vi "PROJECT.vi"() -> ()   [LabVIEW 2020]
uses:
  <vilib>/Utility/file.llb/Read Delimited Spreadsheet (string).vi
  <vilib>/Utility/file.llb/Read Delimited Spreadsheet (DBL).vi
  <vilib>/Utility/file.llb/Write Delimited Spreadsheet (DBL).vi
panel:
  out "TOTAL EVENTS":dbl
  out "USD TO RM":dbl
  out "CRUDE OIL":dbl
  out "TIME":string
  out "DATE":string
  out "EVENT REPORT":string[][](array[string])
  out "INDICATOR":T1
  in  "SECURITY":T2 {"TEMPERATURE" scale=27.0..110.0}
  out "ITEM RECEIVED":bool
  out "PICKUP 4":dbl(slide) scale=0.0..10.0
  out "PROCESSTROLLEYVER 3":dbl(slide)
  out "PICKUP 3":dbl(slide) scale=0.0..10.0
  out "PICKUP 2":dbl(slide) scale=0.0..10.0
  out "PROCESSTROLLEYVER 2":dbl(slide) scale=0.0..10.0
  out "PROCESSTROLLEYVER":dbl(slide) scale=0.0..10.0
  out "BOXVERT":dbl(slide) scale=0.0..10.0
  out "PICKUP":i32(slide) scale=0.0..10.0
  out "TINY":bool
  out "SMALL":bool
  out "MEDIUM":bool
  out "BIG":bool
  out "PRODUCT AVAILABLITY":bool=TRUE
  out "Boolean 2":bool
  out "Boolean":bool
  out "index of element":i32
  out "PRODUCT NOT AVAILABLE":bool
  out "Start":dbl(slide) scale=0.0..10.0
  out "PATH1":dbl(slide) scale=0.0..10.0
  out "PATH7":dbl(slide) scale=0.0..10.0
  out "PATH4":dbl(slide) scale=0.0..10.0
  out "PATH 3":dbl(slide)
  out "PATH9":dbl(slide) scale=0.0..10.0
  out "PATH8":dbl(slide)
  out "PATH2":dbl(slide) scale=0.0..10.0
  out "PATH6":dbl(slide)
  out "PATH5":dbl(slide)
  out "PATH12":dbl(slide) scale=0.0..10.0
  out "PATH11":dbl(slide) scale=0.0..10.0
  out "PATH10":dbl(slide) scale=0.0..10.0
  out "BIG BOX":dbl(slide) scale=0.0..10.0
  out "PACKAGING":dbl(slide) scale=0.0..10.0
  out "x+1":dbl
  out "ALARM":dbl
  out "PROCESSING OFF":bool
  out "login":bool
  out "STRING":string
  out "WEIGHT":string
  out "BOXTYPE":string
  out "ORDER ID":string
  out "all rows":string[](array[string])
  # "MARKET INFORMATION"
  # "AUTOMATED WAREHOUSE MANAGEMENT SYSTEM\n                                                          -NI LABVIEW \n                                                                 -BY ABHISHEK KUMAR JHA"
  # "MEDIUM"
  # "PROCESSING HOUSE"
  # "TINY"
  # "SMALL"
  # "BIG"
  # "SECURITY AND ALARM CENTER"
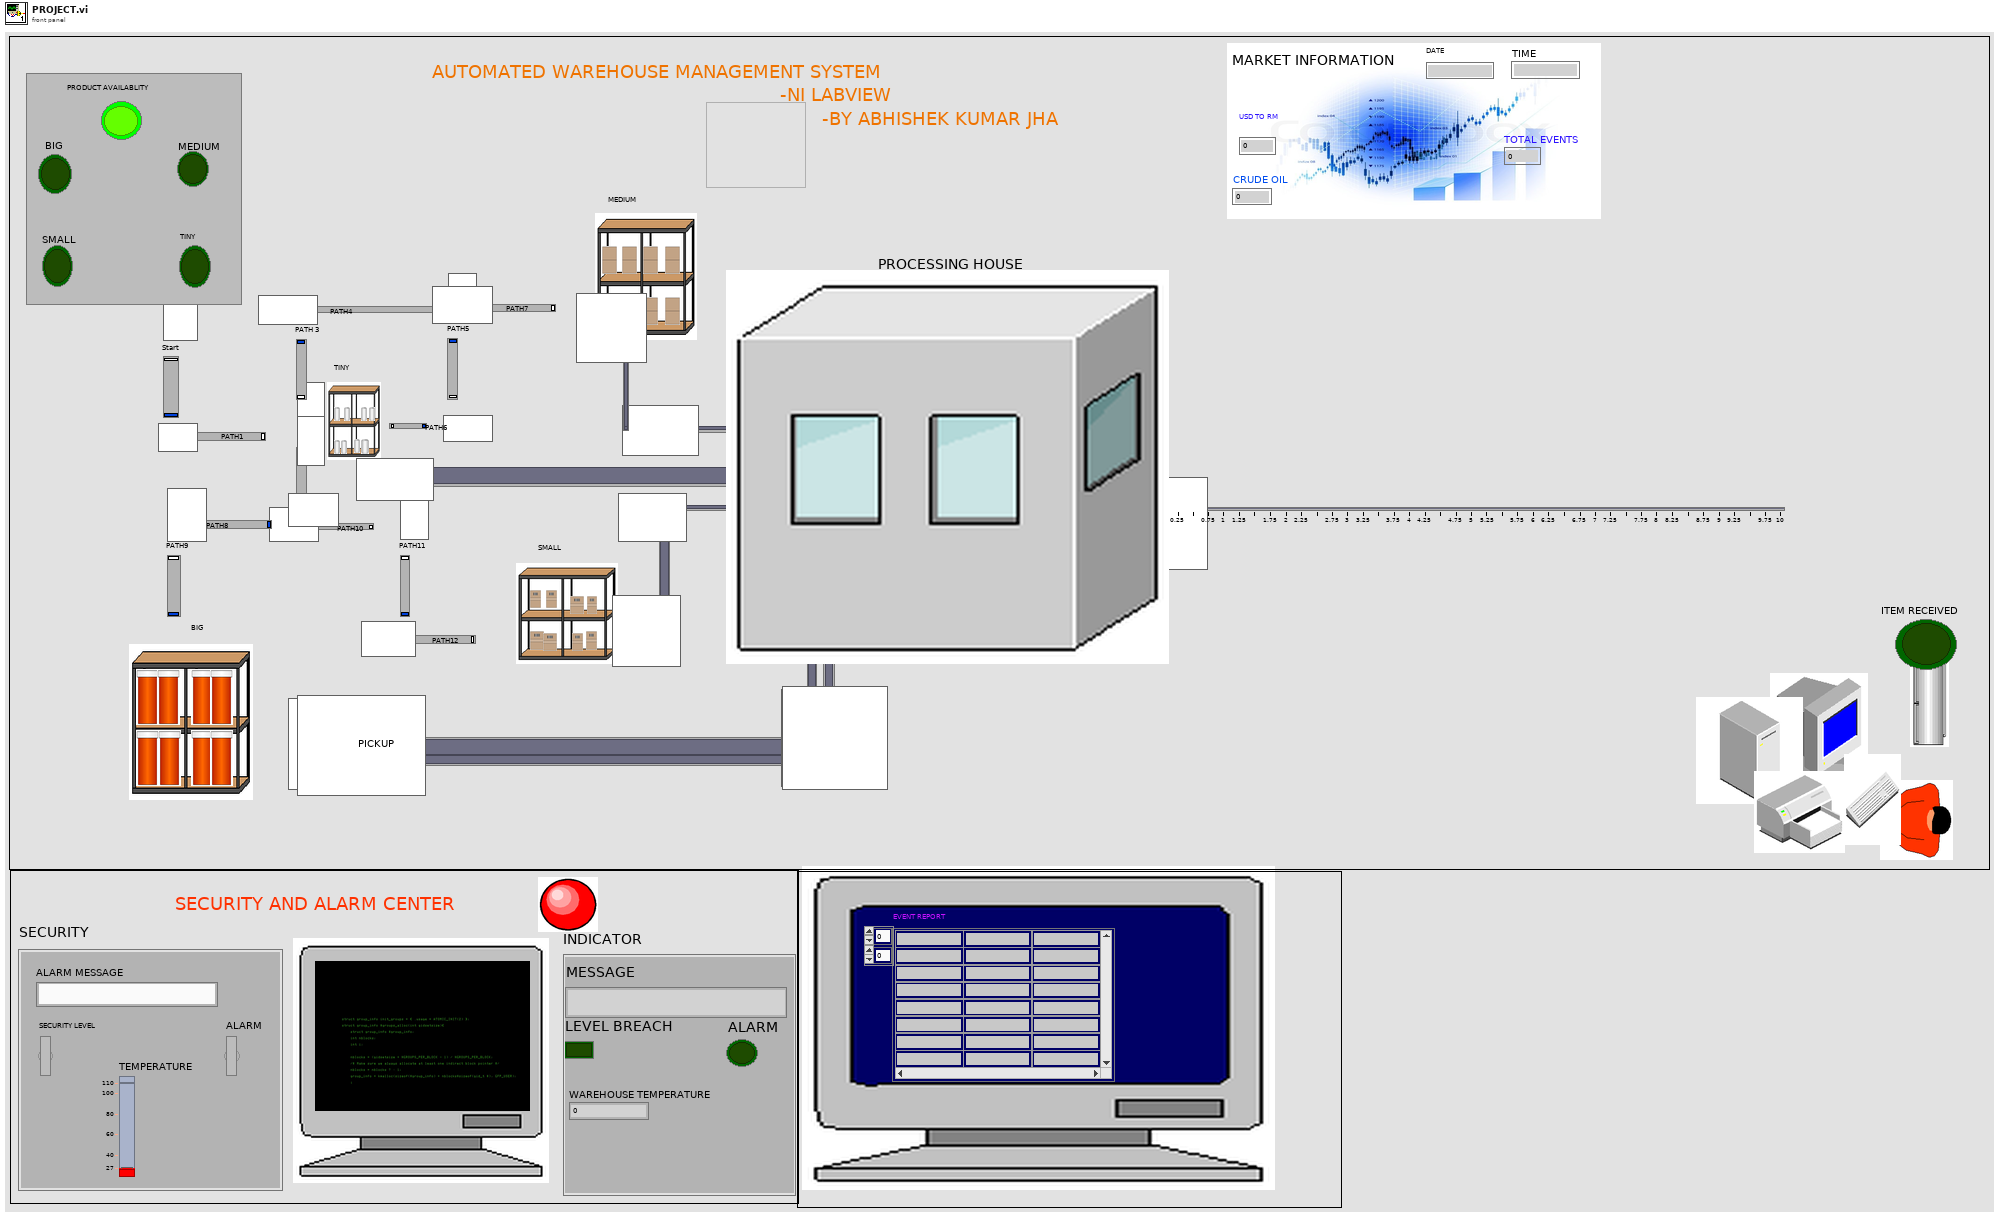
[diagram p1: front panel]
types:
  T1 = cluster{"MESSAGE":string, "LEVEL BREACH":bool, "ALARM":bool, "WAREHOUSE TEMPERATURE":dbl}
  T2 = cluster{"ALARM MESSAGE":string, "SECURITY LEVEL":bool, "ALARM":bool, "TEMPERATURE":dbl}
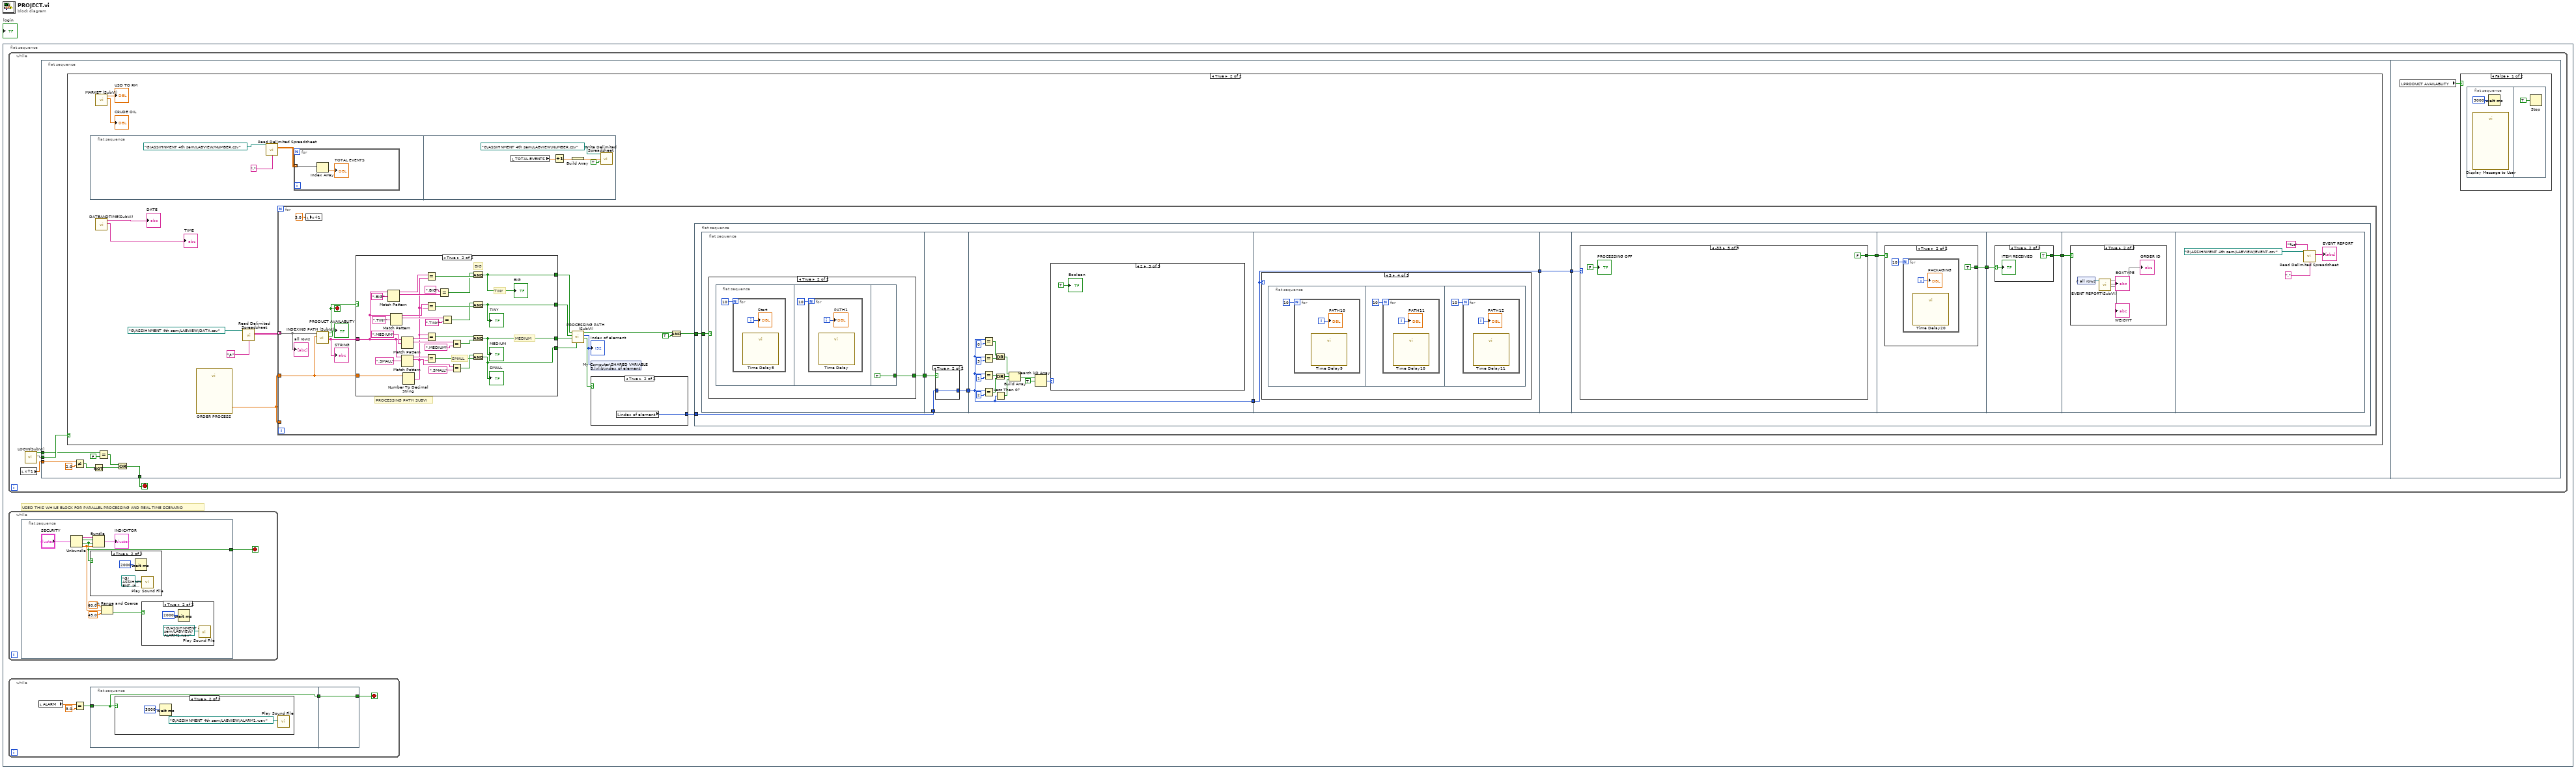
[diagram p0: block diagram]
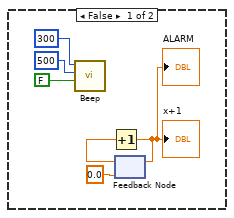
[diagram p5: hidden frame]
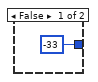
[diagram p6: hidden frame]
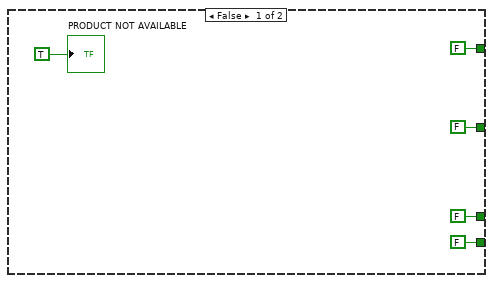
[diagram p7: hidden frame]
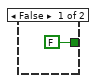
[diagram p8: hidden frame]
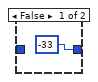
[diagram p9: hidden frame]
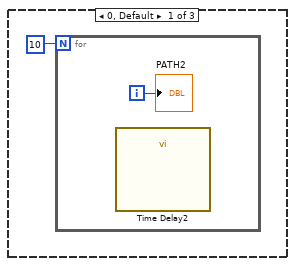
[diagram p10: hidden frame]
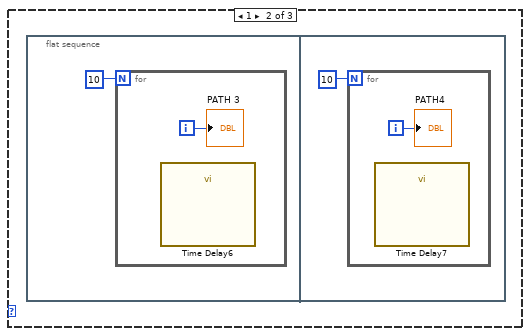
[diagram p11: hidden frame]
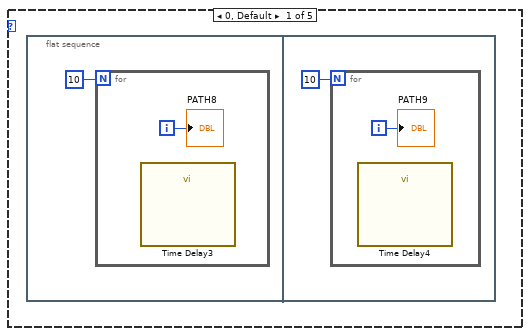
[diagram p12: hidden frame]
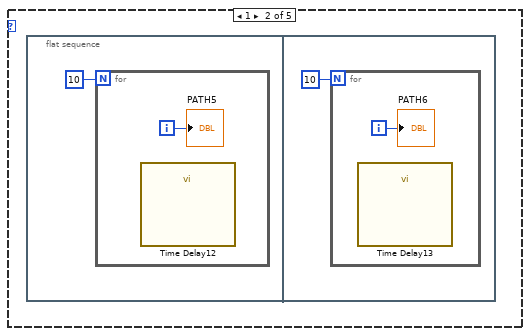
[diagram p13: hidden frame]
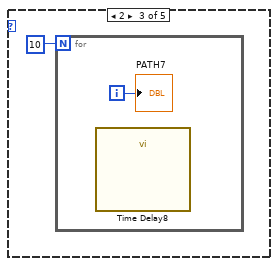
[diagram p14: hidden frame]
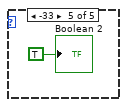
[diagram p15: hidden frame]
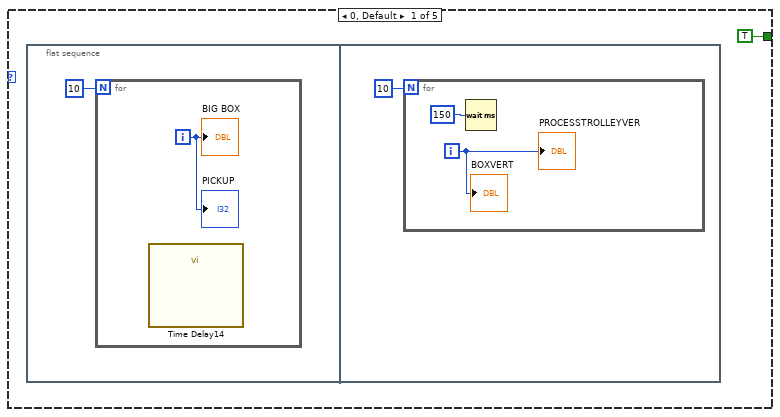
[diagram p16: hidden frame]
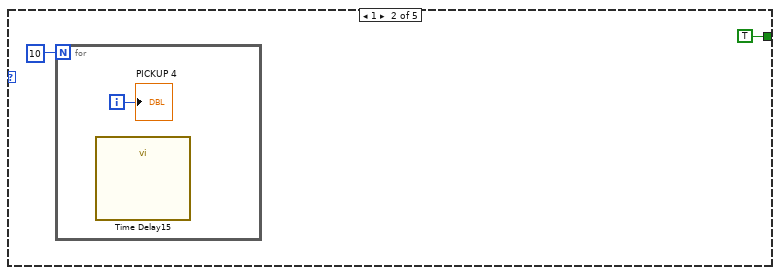
[diagram p17: hidden frame]
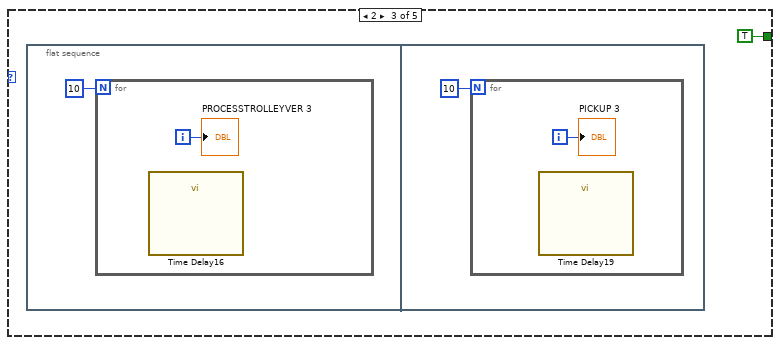
[diagram p18: hidden frame]
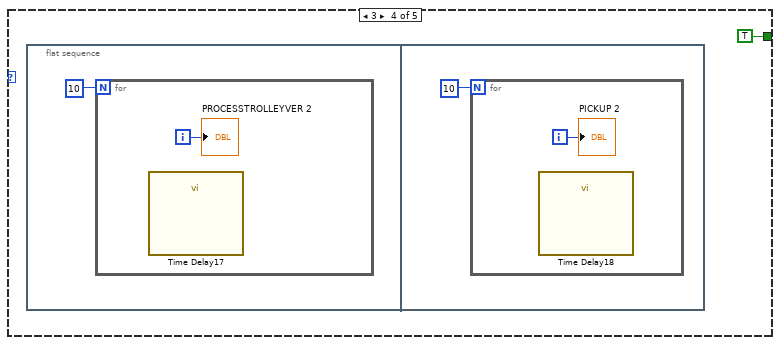
[diagram p19: hidden frame]
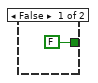
[diagram p20: hidden frame]
diagram:
  n1 = flat-sequence {
    frame #0 {
      # "USED THIS WHILE BLOCK FOR PARALLEL PROCESSING AND REAL TIME SCENARIO"
      n2 = while {
        stop <- w25 stop-if-true
        n3 = local read "x+1"() -> (w27:dbl)
        n4 = call "LOGIN(SubVI).vi"() -> (2:w26, "Boolean"=w24:bool)  [unwired: 10 in]
        n5 = flat-sequence {
          tunnel: w27 -> [w34]
          tunnel: w26 -> [w33]
          tunnel: [w29] -> w25
          tunnel: w24 -> [w28]
          frame #0 {
            n6 = case shown="True" w33 {
              frame False {
                n7 = call <vilib>:"Beep.vi"("use system alert? (T)"=FALSE, "duration (msec)"=u32 500, "frequency (Hz)"=u32 300) -> ()  [unwired: 9 in]
                n8 = feedback #1(0.0) -> (w42:dbl)
                n9 = Increment(x=w42) -> (x+1=w41:dbl)
                "x+1" <- w41
                "ALARM" <- w41
                n10 = feedback-in #1(w41) -> ()
              }
              frame True {
                n11 = flat-sequence {
                  frame #0 {
                    n12 = call-poly <vilib>:"Read Delimited Spreadsheet.vi"("file path (dialog if empty)"=path "G:/ASSIHNMENT 4th sem/LABVIEW/NUMBER.csv", "delimiter (\\t)"="," ("delimiter (\\t)")) -> ("all rows"=w51:dbl[][])  [unwired: 8 in, 5 out]
                    n13 = for {
                      tunnel: w51 -> [w55] mode=indexing
                      n14 = Index Array(array=w55) -> (element=→"TOTAL EVENTS":dbl)  [unwired: 1 in]
                    }
                  }
                  frame #1 {
                    n15 = local read "TOTAL EVENTS"() -> (w57:dbl)
                    n16 = Increment(x=w57) -> (x+1=w56:dbl)
                    n17 = Build Array(w56) -> (w58:dbl[])
                    n18 = call-poly <vilib>:"Write Delimited Spreadsheet.vi"("file path (dialog if empty)"=path "G:/ASSIHNMENT 4th sem/LABVIEW/NUMBER.csv", "1D data"=w58, "append to file? (new file:F)"=TRUE) -> ()  [unwired: 11 in, 2 out]
                  }
                }
                n19 = call "MARKET (SubVI).vi"() -> ("CRUDE OIL"=→"CRUDE OIL":dbl, "USD TO RM"=→"USD TO RM":dbl)  [unwired: 10 in]
                n20 = call "DATEANDTIME(SubVI).vi"() -> ("TIME"=→"TIME":string, "DATE"=→"DATE":string)  [unwired: 10 in]
                n21 = call "ORDER PROCESS"() -> ("ORDER ID:-"=w47:dbl)  [unwired: 17 in, 2 out]
                n22 = call-poly <vilib>:"Read Delimited Spreadsheet.vi"("file path (dialog if empty)"=path "G:/ASSIHNMENT 4th sem/LABVIEW/DATA.csv", "delimiter (\\t)"="\t," ("delimiter (\\t)")) -> ("all rows"=w48:string[][])  [unwired: 8 in, 5 out]
                n23 = for {
                  tunnel: w48 -> [w65] mode=indexing
                  tunnel: w47 -> [w66]
                  tunnel: w47 -> [_]
                  stop <- w75 stop-if-true
                  # "PROCESSING PATH SUBVI"
                  n24 = local write "x+1"(3.0 ("x+1")) -> ()
                  n25 = call "INDEXING PATH (SubVI).vi"("ORDER ID:-"=w66, "ROWS"=w65) -> ("STRING"=w76:string, "PRODUCT AVAILABLITY"=→"PRODUCT AVAILABLITY":bool, "INDIDCATOR"=w75:bool)  [unwired: 7 in]
                  "STRING" <- w76
                  n26 = case shown="True" w75 {
                    tunnel: w66 -> [_ w111]
                    tunnel: w76 -> [_ w88]
                    tunnel: [FALSE ("Boolean 2") w87] -> w74
                    tunnel: [FALSE w86] -> w73
                    tunnel: [FALSE w85] -> w72
                    tunnel: [FALSE w84] -> w71
                    frame False {
                      "PRODUCT NOT AVAILABLE" <- TRUE ("PRODUCT NOT AVAILABLE")
                    }
                    frame True {
                      # "BIG"
                      # "TINY"
                      # "MEDIUM"
                      # "SMALL"
                      n27 = Match Pattern(string=w88, regular expression=",BIG") -> (before substring=w110:string, match substring=w113:string)  [unwired: 1 in, 2 out]
                      n28 = Match Pattern(string=w88, regular expression=",TINY") -> (before substring=w92:string, match substring=w103:string)  [unwired: 1 in, 2 out]
                      n29 = Match Pattern(string=w88, regular expression=",MEDIUM") -> (before substring=w98:string, match substring=w104:string)  [unwired: 1 in, 2 out]
                      n30 = Match Pattern(string=w88, regular expression=",SMALL") -> (before substring=w95:string, match substring=w102:string)  [unwired: 1 in, 2 out]
                      n31 = Number To Decimal String(number=w111) -> (decimal integer string=w91:string)  [unwired: 1 in]
                      n32 = Equal?(x=w110, y=w91) -> (x = y?=w109:bool)
                      n33 = Equal?(x=w92, y=w91) -> (x = y?=w90:bool)
                      n34 = Equal?(x=w91, y=w98) -> (x = y?=w97:bool)
                      n35 = Equal?(x=w95, y=w91) -> (x = y?=w94:bool)
                      n36 = Equal?(x=",BIG", y=w113) -> (x = y?=w108:bool)
                      n37 = Equal?(x=w103, y=",TINY") -> (x = y?=w89:bool)
                      n38 = Equal?(x=w104, y=",MEDIUM") -> (x = y?=w96:bool)
                      n39 = Equal?(x=w102, y=",SMALL") -> (x = y?=w93:bool)
                      n40 = And(x=w108, y=w109) -> (x .and. y?=w87:bool)
                      "BIG" <- w87
                      n41 = And(x=w89, y=w90) -> (x .and. y?=w86:bool)
                      "TINY" <- w86
                      n42 = And(x=w97, y=w96) -> (x .and. y?=w85:bool)
                      "MEDIUM" <- w85
                      n43 = And(x=w93, y=w94) -> (x .and. y?=w84:bool)
                      "SMALL" <- w84
                    }
                  }
                  n44 = call "PROCESSING PATH (SubVI).vi"("Boolean 3"=w71, "Boolean 4"=w72, "Boolean 5"=w73, "Boolean 6"=w74) -> ("Boolean"=w64:bool, "index of element"=w63:i32, "Boolean 2"=w68:bool)  [unwired: 5 in]
                  "index of element" <- w63
                  n45 = shared-variable "My Computer\\SHARED VARIABLE 3.lvlib\\index of element"(w63) -> ()  [unwired: 1 in, 1 out]
                  n46 = case shown="True" w64 {
                    tunnel: [-33 w78] -> w67
                    frame False {
                    }
                    frame True {
                      n47 = local read "index of element"() -> (w78:i32)
                    }
                  }
                  n48 = And(x=w68, y=TRUE) -> (x .and. y?=w69:bool)
                  n49 = flat-sequence {
                    tunnel: w69 -> [w122]
                    tunnel: w67 -> [w120]
                    frame #0 {
                      n50 = flat-sequence {
                        tunnel: w122 -> [w126]
                        tunnel: [w125] -> w121
                        tunnel: [w136] -> w123
                        tunnel: w121 -> [w135]
                        tunnel: w120 -> [w134]
                        tunnel: [w139] -> w124
                        tunnel: w123 -> [w139]
                        tunnel: w124 -> [w161]
                        tunnel: [w161] -> w118
                        tunnel: [w179] -> w119
                        tunnel: w118 -> [w179]
                        tunnel: w119 -> [w181]
                        tunnel: [w180] -> w117
                        tunnel: w117 -> [w204]
                        tunnel: [w203] -> w116
                        tunnel: w116 -> [w209]
                        tunnel: [w210] -> w115
                        tunnel: w115 -> [w214]
                        frame #0 {
                          n51 = case shown="True" w126 {
                            tunnel: [FALSE w128] -> w125
                            frame False {
                            }
                            frame True {
                              n52 = flat-sequence {
                                tunnel: [TRUE] -> w128
                                frame #0 {
                                n53 = for {
                                N: 10 -> [_]
                                i -> [w130]
                                n54 = call "Time Delay5"() -> ()  [unwired: 11 in, 1 out]
                                "Start" <- w130
                                }
                                }
                                frame #1 {
                                n55 = for {
                                N: 10 -> [_]
                                i -> [w132]
                                n56 = call "Time Delay"() -> ()  [unwired: 11 in, 1 out]
                                "PATH1" <- w132
                                }
                                }
                                frame #2 {
                                }
                              }
                            }
                          }
                        }
                        frame #1 {
                          n57 = case shown="True" w135 {
                            tunnel: [-33 w138] -> w136
                            tunnel: w134 -> [_ w138]
                            frame False {
                            }
                            frame True {
                            }
                          }
                        }
                        frame #2 {
                          n58 = Equal?(x=w139, y=0) -> (x = y?=w151:bool)
                          n59 = Equal?(x=w139, y=3) -> (x = y?=w150:bool)
                          n60 = Equal?(x=w139, y=1) -> (x = y?=w147:bool)
                          n61 = Equal?(x=w139, y=2) -> (x = y?=w146:bool)
                          n62 = Or(x=w151, y=w150) -> (x .or. y?=w145:bool)
                          n63 = Or(x=w147, y=w146) -> (x .or. y?=w144:bool)
                          n64 = Less Than 0?(x=w139) -> (x < 0?=w143:bool)
                          n65 = Build Array(w145, w144, w143) -> (w142:bool[])
                          n66 = Search 1D Array(1D array=w142, element=TRUE) -> (index of element=w140:i32)  [unwired: 1 in]
                          n67 = case shown="2" w140 {
                            frame 0, Default {
                              n68 = for {
                                N: 10 -> [_]
                                i -> [w155]
                                n69 = call "Time Delay2"() -> ()  [unwired: 11 in, 1 out]
                                "PATH2" <- w155
                              }
                            }
                            frame 1 {
                              n70 = flat-sequence {
                                frame #0 {
                                n71 = for {
                                N: 10 -> [_]
                                i -> [w157]
                                n72 = call "Time Delay6"() -> ()  [unwired: 11 in, 1 out]
                                "PATH 3" <- w157
                                }
                                }
                                frame #1 {
                                n73 = for {
                                N: 10 -> [_]
                                i -> [w159]
                                n74 = call "Time Delay7"() -> ()  [unwired: 11 in, 1 out]
                                "PATH4" <- w159
                                }
                                }
                              }
                            }
                            frame 2 {
                              "Boolean" <- TRUE
                            }
                          }
                        }
                        frame #3 {
                          n75 = case shown="3" w161 {
                            frame 0, Default {
                              n76 = flat-sequence {
                                frame #0 {
                                n77 = for {
                                N: 10 -> [_]
                                i -> [w163]
                                n78 = call "Time Delay3"() -> ()  [unwired: 11 in, 1 out]
                                "PATH8" <- w163
                                }
                                }
                                frame #1 {
                                n79 = for {
                                N: 10 -> [_]
                                i -> [w165]
                                n80 = call "Time Delay4"() -> ()  [unwired: 11 in, 1 out]
                                "PATH9" <- w165
                                }
                                }
                              }
                            }
                            frame 1 {
                              n81 = flat-sequence {
                                frame #0 {
                                n82 = for {
                                N: 10 -> [_]
                                i -> [w167]
                                n83 = call "Time Delay12"() -> ()  [unwired: 11 in, 1 out]
                                "PATH5" <- w167
                                }
                                }
                                frame #1 {
                                n84 = for {
                                N: 10 -> [_]
                                i -> [w169]
                                n85 = call "Time Delay13"() -> ()  [unwired: 11 in, 1 out]
                                "PATH6" <- w169
                                }
                                }
                              }
                            }
                            frame 2 {
                              n86 = for {
                                N: 10 -> [_]
                                i -> [w171]
                                n87 = call "Time Delay8"() -> ()  [unwired: 11 in, 1 out]
                                "PATH7" <- w171
                              }
                            }
                            frame 3 {
                              n88 = flat-sequence {
                                frame #0 {
                                n89 = for {
                                N: 10 -> [_]
                                i -> [w173]
                                n90 = call "Time Delay9"() -> ()  [unwired: 11 in, 1 out]
                                "PATH10" <- w173
                                }
                                }
                                frame #1 {
                                n91 = for {
                                N: 10 -> [_]
                                i -> [w175]
                                n92 = call "Time Delay10"() -> ()  [unwired: 11 in, 1 out]
                                "PATH11" <- w175
                                }
                                }
                                frame #2 {
                                n93 = for {
                                N: 10 -> [_]
                                i -> [w177]
                                n94 = call "Time Delay11"() -> ()  [unwired: 11 in, 1 out]
                                "PATH12" <- w177
                                }
                                }
                              }
                            }
                            frame -33 {
                              "Boolean 2" <- TRUE
                            }
                          }
                        }
                        frame #4 {
                        }
                        frame #5 {
                          n95 = case shown="-33" w181 {
                            tunnel: [TRUE TRUE TRUE TRUE FALSE] -> w180
                            frame 0, Default {
                              n96 = flat-sequence {
                                frame #0 {
                                n97 = for {
                                N: 10 -> [_]
                                i -> [w184]
                                n98 = call "Time Delay14"() -> ()  [unwired: 11 in, 1 out]
                                "PICKUP" <- w184
                                "BIG BOX" <- w184
                                }
                                }
                                frame #1 {
                                n99 = for {
                                N: 10 -> [_]
                                i -> [w187]
                                n100 = Wait (ms)(milliseconds to wait=u32 150) -> ()  [unwired: 1 out]
                                "BOXVERT" <- w187
                                "PROCESSTROLLEYVER" <- w187
                                }
                                }
                              }
                            }
                            frame 1 {
                              n101 = for {
                                N: 10 -> [_]
                                i -> [w190]
                                n102 = call "Time Delay15"() -> ()  [unwired: 11 in, 1 out]
                                "PICKUP 4" <- w190
                              }
                            }
                            frame 2 {
                              n103 = flat-sequence {
                                frame #0 {
                                n104 = for {
                                N: 10 -> [_]
                                i -> [w193]
                                n105 = call "Time Delay16"() -> ()  [unwired: 11 in, 1 out]
                                "PROCESSTROLLEYVER 3" <- w193
                                }
                                }
                                frame #1 {
                                n106 = for {
                                N: 10 -> [_]
                                i -> [w195]
                                n107 = call "Time Delay19"() -> ()  [unwired: 11 in, 1 out]
                                "PICKUP 3" <- w195
                                }
                                }
                              }
                            }
                            frame 3 {
                              n108 = flat-sequence {
                                frame #0 {
                                n109 = for {
                                N: 10 -> [_]
                                i -> [w198]
                                n110 = call "Time Delay17"() -> ()  [unwired: 11 in, 1 out]
                                "PROCESSTROLLEYVER 2" <- w198
                                }
                                }
                                frame #1 {
                                n111 = for {
                                N: 10 -> [_]
                                i -> [w200]
                                n112 = call "Time Delay18"() -> ()  [unwired: 11 in, 1 out]
                                "PICKUP 2" <- w200
                                }
                                }
                              }
                            }
                            frame -33 {
                              "PROCESSING OFF" <- FALSE
                            }
                          }
                        }
                        frame #6 {
                          n113 = case shown="True" w204 {
                            tunnel: [FALSE TRUE] -> w203
                            frame False {
                            }
                            frame True {
                              n114 = for {
                                N: 10 -> [_]
                                i -> [w208]
                                n115 = call "Time Delay20"() -> ()  [unwired: 11 in, 1 out]
                                "PACKAGING" <- w208
                              }
                            }
                          }
                        }
                        frame #7 {
                          n116 = case shown="True" w209 {
                            selector: w209 -> [_ w212]
                            tunnel: [FALSE TRUE] -> w210
                            frame False {
                            }
                            frame True {
                              "ITEM RECEIVED" <- w212
                            }
                          }
                        }
                        frame #8 {
                          n117 = case shown="True" w214 {
                            frame False {
                            }
                            frame True {
                              n118 = control-ref of="all rows"() -> (w218:refnum<vi>)
                              n119 = call "EVENT REPORT(SubVI).vi"("ORDER ID:-"=w218) -> (1:→"WEIGHT", 2:→"BOXTYPE", 3:→"ORDER ID")  [unwired: 8 in]
                            }
                          }
                        }
                        frame #9 {
                          n120 = call-poly <vilib>:"Read Delimited Spreadsheet.vi"("file path (dialog if empty)"=path "G:/ASSIHNMENT 4th sem/LABVIEW/EVENT.csv", "format (%s)"="%s", "delimiter (\\t)"="," ("delimiter (\\t)")) -> ("all rows"=→"EVENT REPORT":string[][])  [unwired: 7 in, 5 out]
                        }
                      }
                    }
                  }
                  "all rows" <- w65
                }
              }
            }
            n121 = Not Equal?(x=w34, y=2.0) -> (x != y?=w35:bool)
            n122 = Not(x=w35) -> (.not. x?=w30:bool)
            n123 = Equal?(x=w28, y=FALSE) -> (x = y?=w31:bool)
            n124 = Or(x=w31, y=w30) -> (x .or. y?=w29:bool)
          }
          frame #1 {
            n125 = local read "PRODUCT AVAILABLITY"() -> (w223:bool)
            n126 = case shown="False" w223 {
              frame False {
                n127 = flat-sequence {
                  frame #0 {
                    n128 = call "Display Message to User"() -> ()  [unwired: 10 in, 2 out]
                    n129 = Wait (ms)(milliseconds to wait=u32 3000) -> ()  [unwired: 1 out]
                  }
                  frame #1 {
                    n130 = Stop(stop? (T)=TRUE) -> ()
                  }
                }
              }
              frame True {
              }
            }
          }
        }
      }
      n131 = while {
        stop <- w10 stop-if-true
        n132 = flat-sequence {
          tunnel: [w11] -> w10
          frame #0 {
            n133 = Unbundle("SECURITY") -> ("ALARM MESSAGE"=w18:string, "SECURITY LEVEL"=w16:bool, "ALARM"=w11:bool, "TEMPERATURE"=w15:dbl)
            n134 = case shown="True" w11 {
              frame False {
              }
              frame True {
                n135 = Wait (ms)(milliseconds to wait=u32 2000) -> ()  [unwired: 1 out]
                n136 = call <vilib>:"Play Sound File.vi"("path"=path "G:/ASSIHNMENT 4th sem/LABVIEW/ALARM1.wav") -> ()  [unwired: 9 in, 2 out]
              }
            }
            n137 = Bundle("ALARM MESSAGE"=w18, "SECURITY LEVEL"=w16, "ALARM"=w11, "TEMPERATURE"=w15) -> (→"INDICATOR":T2)  [unwired: 1 in]
            n138 = In Range and Coerce(upper limit=60.0, x=w15, lower limit=45.0) -> (In Range?=w12:bool)  [unwired: 1 out]
            n139 = case shown="True" w12 {
              frame False {
              }
              frame True {
                n140 = Wait (ms)(milliseconds to wait=u32 2000) -> ()  [unwired: 1 out]
                n141 = call <vilib>:"Play Sound File.vi"("path"=path "G:/ASSIHNMENT 4th sem/LABVIEW/ALARM1.wav") -> ()  [unwired: 9 in, 2 out]
              }
            }
          }
        }
      }
      n142 = while {
        stop <- w1 stop-if-true
        n143 = local read "ALARM"() -> (w5:dbl)
        n144 = Equal?(x=w5, y=3.0) -> (x = y?=w3:bool)
        n145 = flat-sequence {
          tunnel: w3 -> [w6]
          tunnel: [w6] -> w2
          tunnel: w2 -> [w9]
          tunnel: [w9] -> w1
          frame #0 {
            n146 = case shown="True" w6 {
              frame False {
              }
              frame True {
                n147 = Wait (ms)(milliseconds to wait=u32 3000) -> ()  [unwired: 1 out]
                n148 = call <vilib>:"Play Sound File.vi"("path"=path "G:/ASSIHNMENT 4th sem/LABVIEW/ALARM1.wav") -> ()  [unwired: 9 in, 2 out]
              }
            }
          }
          frame #1 {
          }
        }
      }
    }
  }
